vi "SnapAndParthing.vi"(10 "ResultIN":string[][](array[string]), 11 "Vision&Robot":refnum<vi>) -> (2 "Name":string[](array[string]), 3 "OK/NG":bool)   [LabVIEW 2019]
uses:
  VisionSet/System/iVision/Controls/Parameter.ctl
panel:
  # "P_X_1"
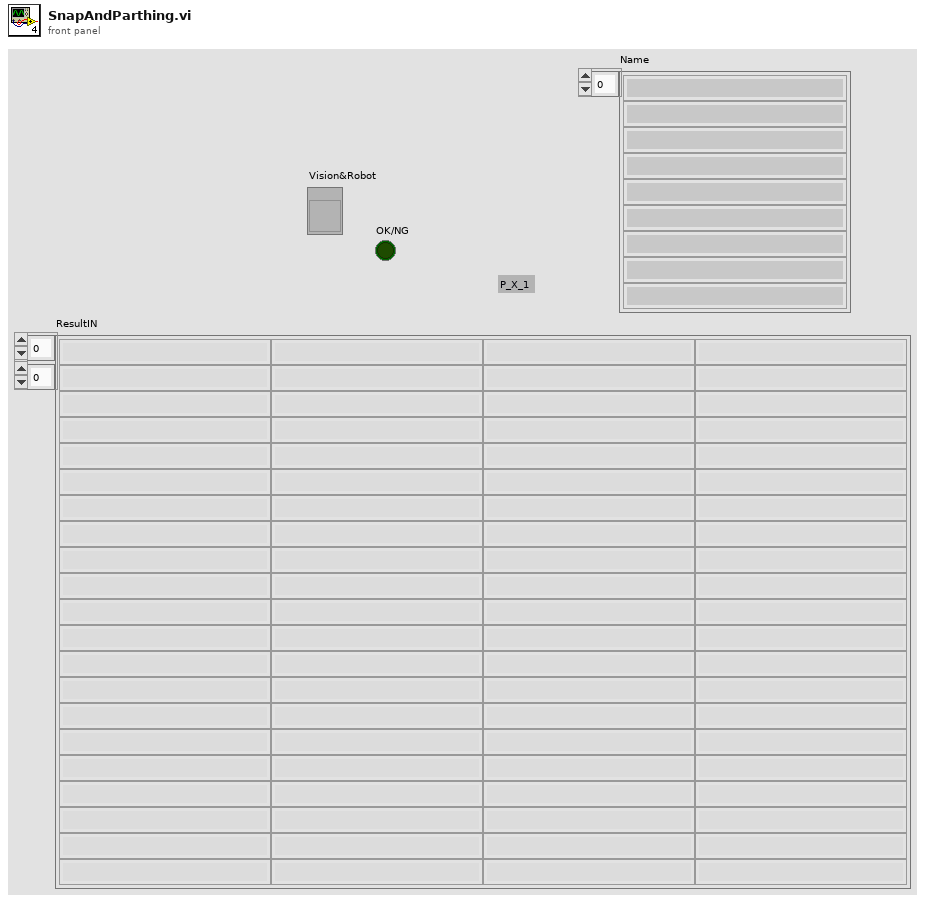
[diagram p1: front panel]
types:
  T1 = typedef "Parameter.ctl" = enum16{"Initialize", "Write", "Read", "WriteAll", "Save", "Load"}
  T2 = typedef "ParameterData.ctl" = cluster{"Rotate Angle":dbl, "Rotate?":bool, "Calibration File Path":string, "Cal?":bool}
  T3 = cluster{"VisionPoint":cluster{"X":dbl, "Y":dbl}, "RobotPoint":cluster{"X":dbl, "Y":dbl, "U":dbl}}[]
  T4 = cluster{"VisionPoint":cluster{"X":dbl, "Y":dbl}, "RobotPoint":cluster{"X":dbl, "Y":dbl, "U":dbl}}
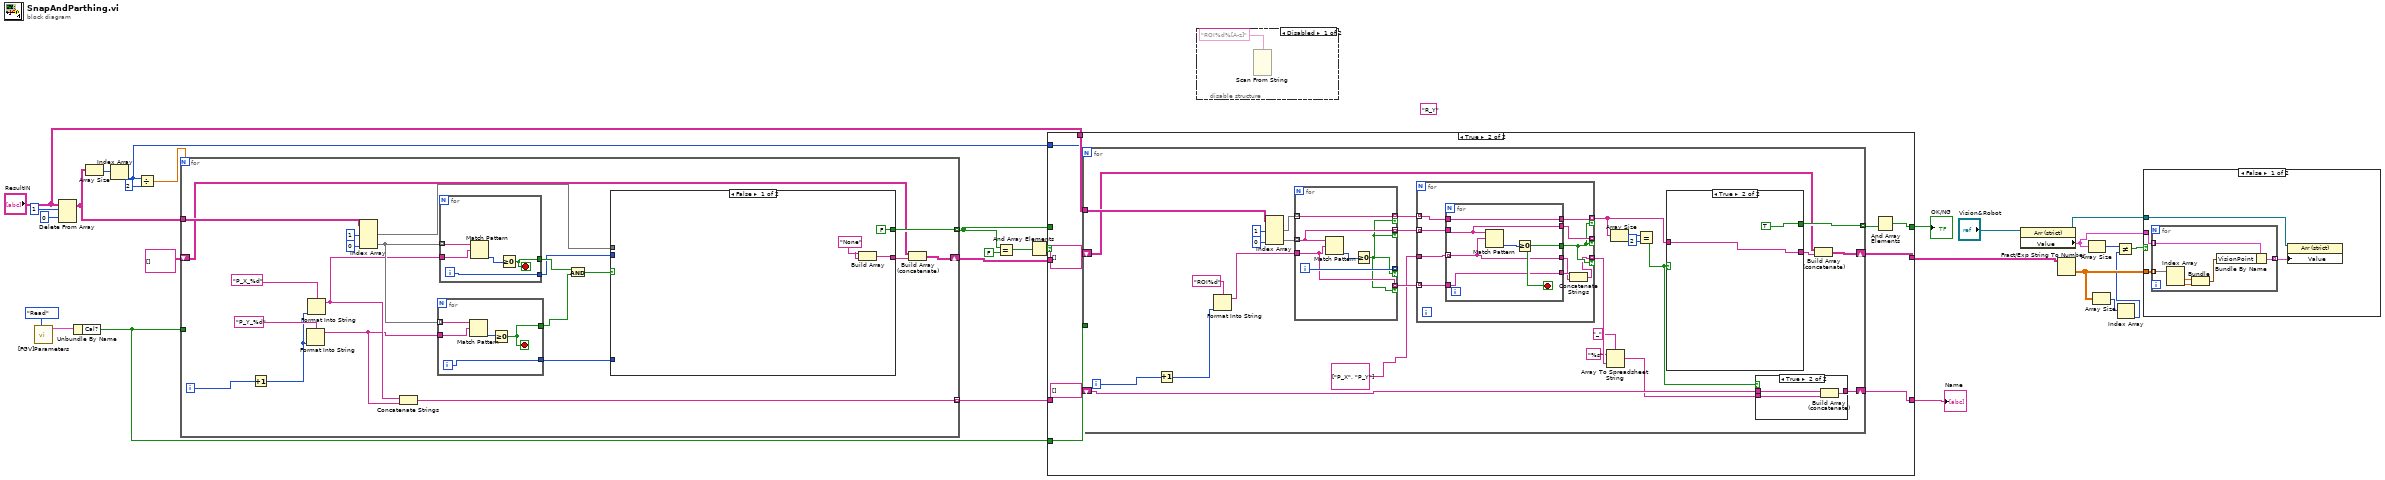
[diagram p0: block diagram]
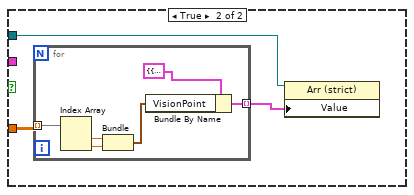
[diagram p2: hidden frame]
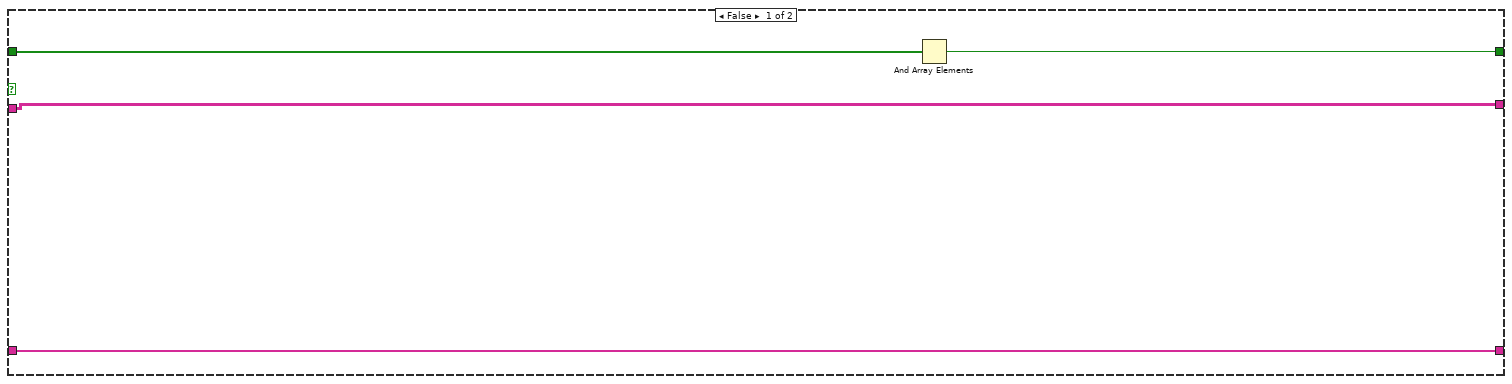
[diagram p4: hidden frame]
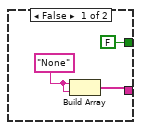
[diagram p6: hidden frame]
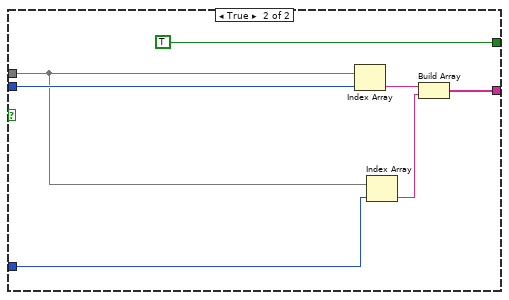
[diagram p7: hidden frame]
diagram:
  (unwired) "R_Y"
  n1 = call "[FGV]Parameters.vi"("Parameter"=Parameter."Read") -> ("ParameterData Out"=w27:T2)  [unwired: 9 in, 1 out]
  n2 = Delete From Array(array="ResultIN", length=1, index (row)=0) -> (array with subset deleted=w1:string[][])  [unwired: 1 in, 1 out]
  n3 = Unbundle By Name(w27) -> ("Cal?"=w12:bool)
  n4 = Array Size(array=w1) -> (size(s)=w25:i32[])
  n5 = Index Array(array=w25) -> (element=w9:i32)  [unwired: 1 in]
  n6 = Divide(x=w9, y=2) -> (x/y=w13:dbl)
  n7 = for {
    N: w13 -> [_]
    tunnel: w1 -> [w46]
    tunnel: w12 -> [_]
    tunnel: [w34] -> w14 mode=indexing
    tunnel: [w33] -> w17 mode=indexing
    shift-right: [w31] -> w10
    shift-left: string[][] [] -> [w30]
    i -> [w48]
    n8 = Increment(x=w48) -> (x+1=w47:i32)
    n9 = Format Into String(format string="P_Y_%d", w47) -> (resulting string=w35:string)  [unwired: 2 in, 1 out]
    n10 = Format Into String(format string="P_X_%d", w47) -> (resulting string=w36:string)  [unwired: 2 in, 1 out]
    n11 = Index Array(array=w46, index (col) #1=1 ("disabled index (col)"), index (col) #2=0 ("disabled index (col)")) -> (element #1=w42:string[], element #2=w44:string[])  [unwired: 2 in]
    n12 = Concatenate Strings(w36, w35) -> (w34:string)
    n13 = for {
      tunnel: w44 -> [w65] mode=indexing
      tunnel: w35 -> [w64]
      tunnel: [w62] -> w40
      tunnel: [w61] -> w37
      i -> [w61]
      stop <- w62 stop-if-true
      n14 = Match Pattern(string=w65, regular expression=w64) -> (offset past match=w63:i32)  [unwired: 1 in, 3 out]
      n15 = Greater Or Equal To 0?(x=w63) -> (x >= 0?=w62:bool)
    }
    n16 = for {
      tunnel: w44 -> [w70] mode=indexing
      tunnel: w36 -> [w69]
      tunnel: [w67] -> w41
      tunnel: [w66] -> w39
      i -> [w66]
      stop <- w67 stop-if-true
      n17 = Match Pattern(string=w70, regular expression=w69) -> (offset past match=w68:i32)  [unwired: 1 in, 3 out]
      n18 = Greater Or Equal To 0?(x=w68) -> (x >= 0?=w67:bool)
    }
    n19 = And(x=w41, y=w40) -> (x .and. y?=w38:bool)
    n20 = case shown="False" w38 {
      tunnel: w42 -> [_ w59]
      tunnel: w39 -> [_ w60]
      tunnel: w37 -> [_ w58]
      tunnel: [FALSE TRUE] -> w33
      tunnel: [w52 w54] -> w32
      frame False {
        w51 = "None"
        n21 = Build Array(w51, w51) -> (w52:string[])
      }
      frame True {
        n22 = Index Array(array=w59, index=w60) -> (element=w57:string)
        n23 = Index Array(array=w59, index=w58) -> (element=w56:string)
        n24 = Build Array(w57, w56) -> (w54:string[])
      }
    }
    n25 = Build Array (concatenate)(w30, w32) -> (w31:string[][])
  }
  n26 = Equal?(x=w17, y=FALSE) -> (x = y?=w19:bool[])
  n27 = And Array Elements(Boolean array=w19) -> (logical AND=w18:bool)
  n28 = case shown="True" w18 {
    tunnel: w17 -> [w74 _]
    tunnel: [w73 w76] -> w16
    tunnel: [w72 w79] -> w15
    tunnel: w14 -> [w72 _]
    tunnel: "ResultIN" -> [_ w82]
    tunnel: w12 -> [_ w81]
    tunnel: [w71 w80] -> w11
    tunnel: w10 -> [w71 _]
    tunnel: w9 -> [_ w75]
    frame False {
      n29 = And Array Elements(Boolean array=w74) -> (logical AND=w73:bool)
    }
    frame True {
      n30 = for {
        N: w75 -> [_]
        tunnel: w82 -> [w107]
        tunnel: w81 -> [_]
        tunnel: [w102] -> w77 mode=indexing
        shift-right: [w100] -> w80
        shift-left: string[][] [] -> [w99]
        shift-right: [w92] -> w79
        shift-left: string[] [] -> [w90]
        i -> [w109]
        n31 = Increment(x=w109) -> (x+1=w108:i32)
        n32 = Format Into String(format string="ROI%d", w108) -> (resulting string=w103:string)  [unwired: 2 in, 1 out]
        n33 = Index Array(array=w107, index (col) #1=1 ("disabled index (col)"), index (col) #2=0 ("disabled index (col)")) -> (element #1=w98:string[], element #2=w105:string[])  [unwired: 2 in]
        n34 = for {
          tunnel: w105 -> [w140] mode=indexing
          tunnel: w103 -> [w137]
          tunnel: [w140] -> w97 mode=indexing if=w136
          tunnel: [w139] -> _ mode=indexing if=w136
          tunnel: w98 -> [w138] mode=indexing
          tunnel: [w138] -> w96 mode=indexing if=w136
          tunnel: [w137] -> w91 mode=indexing if=w136
          i -> [w139]
          n35 = Match Pattern(string=w140, regular expression=w137) -> (offset past match=w141:i32)  [unwired: 1 in, 3 out]
          n36 = Greater Or Equal To 0?(x=w141) -> (x >= 0?=w136:bool)
        }
        n37 = for {
          tunnel: w97 -> [w124] mode=indexing
          tunnel: string[] ["P_X", "P_Y"] -> [w123]
          tunnel: w96 -> [w122] mode=indexing
          tunnel: [w121] -> w93 mode=indexing if=w119
          tunnel: [w120] -> _ mode=indexing if=w119
          tunnel: [w115] -> w89 mode=indexing if=w119
          tunnel: w91 -> [w118] mode=indexing
          n38 = for {
            tunnel: w124 -> [w127]
            tunnel: w123 -> [w126] mode=indexing
            tunnel: w122 -> [w129]
            tunnel: [w129] -> w121
            tunnel: [w128] -> w119
            tunnel: [w127] -> w120
            tunnel: [w126] -> w116
            tunnel: w118 -> [w125]
            tunnel: [w125] -> w117
            stop <- w128 stop-if-true
            n39 = Match Pattern(string=w127, regular expression=w126) -> (offset past match=w130:i32)  [unwired: 1 in, 3 out]
            n40 = Greater Or Equal To 0?(x=w130) -> (x >= 0?=w128:bool)
          }
          n41 = Concatenate Strings(w117, w116) -> (w115:string)
        }
        n42 = Array To Spreadsheet String(delimiter (Tab)="_", array=w89, 3:"%s" ("format string")) -> (spreadsheet string=w87:string)
        n43 = Array Size(array=w93) -> (size(s)=w95:i32)
        n44 = Equal?(x=w95, y=2) -> (x = y?=w85:bool)
        n45 = case shown="True" w85 {
          tunnel: w93 -> [_ w134]
          tunnel: [FALSE TRUE] -> w102
          tunnel: [w132 w134] -> w101
          frame False {
            w131 = "None"
            n46 = Build Array(w131, w131) -> (w132:string[])
          }
          frame True {
          }
        }
        n47 = case shown="True" w85 {
          tunnel: [w111 w114] -> w92
          tunnel: w90 -> [w111 w113]
          tunnel: w87 -> [_ w112]
          frame False {
          }
          frame True {
            n48 = Build Array (concatenate)(w113, w112) -> (w114:string[])
          }
        }
        n49 = Build Array (concatenate)(w99, w101) -> (w100:string[][])
      }
      n50 = And Array Elements(Boolean array=w77) -> (logical AND=w76:bool)
    }
  }
  "Name" <- w15
  "OK/NG" <- w16
  n51 = disable-structure shown="Disabled" {
    frame Disabled {
      n52 = Scan From String(format string="ROI%d%[A-z]") -> ()  [unwired: 7 in, 3 out]
    }
    frame Enabled {
    }
  }
  n53 = property class="Arr (strict)"(reference="Vision&Robot") -> (reference out=w22:refnum<vi>, "Value"=w3:T3)  [unwired: 1 in, 1 out]
  n54 = Fract/Exp String To Number(string=w11) -> (number=w7:dbl[][])  [unwired: 3 in, 1 out]
  n55 = Array Size(array=w3) -> (size(s)=w8:i32)
  n56 = Array Size(array=w7) -> (size(s)=w5:i32[])
  n57 = Index Array(array=w5) -> (element=w4:i32)  [unwired: 1 in]
  n58 = Not Equal?(x=w8, y=w4) -> (x != y?=w6:bool)
  n59 = case shown="False" w6 {
    tunnel: w22 -> [w146 w155]
    tunnel: w7 -> [w144 w153]
    tunnel: w3 -> [w143 _]
    frame False {
      n60 = for {
        tunnel: w143 -> [w152] mode=indexing
        tunnel: [w151] -> w145 mode=indexing
        tunnel: w144 -> [w150] mode=indexing
        n61 = Index Array(array=w150) -> (element #1=w149:dbl, element #2=w148:dbl)  [unwired: 2 in]
        n62 = Bundle("Score"=w149, "Score"=w148) -> (w147:cluster{"Score":dbl, "Score":dbl})  [unwired: 1 in]
        n63 = Bundle By Name(cluster=w152, "VisionPoint"=w147) -> (w151:T4)
      }
      n64 = property class="Arr (strict)"(reference=w146, "Value"=w145) -> ()  [unwired: 1 in, 2 out]
    }
    frame True {
      n65 = for {
        tunnel: [w161] -> w154 mode=indexing
        tunnel: w153 -> [w160] mode=indexing
        n66 = Index Array(array=w160) -> (element #1=w159:dbl, element #2=w158:dbl)  [unwired: 2 in]
        n67 = Bundle("Score"=w159, "Score"=w158) -> (w157:cluster{"Score":dbl, "Score":dbl})  [unwired: 1 in]
        n68 = Bundle By Name(cluster=T4 {"VisionPoint"={"X"=0.0, "Y"=0.0}, "RobotPoint"={"X"=0.0, "Y"=0.0, "U"=0.0}} ("Data"), "VisionPoint"=w157) -> (w161:T4)
      }
      n69 = property class="Arr (strict)"(reference=w155, "Value"=w154) -> ()  [unwired: 1 in, 2 out]
    }
  }
